vi "Configure DC Input Resistance.vi"(8 "error in (no error)":errorcluster, 10 "DC Input Resistance Mode (0: Fixed)":u16(ring) items=["Fixed", "Auto"], 11 "VISA resource name":refnum<visa-resource-name>) -> (0 "error out":errorcluster, 3 "VISA resource name out":refnum<visa-resource-name>)   [LabVIEW 2020, in "Agilent 34401.lvlib"]
doc: "Sets the input resistance for voltage readings."
uses:
  <instrlib>/Agilent 34401/Agilent 34401.lvlib
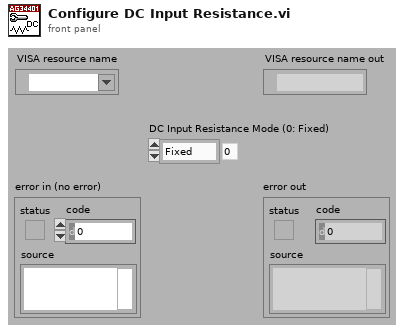
[diagram p1: front panel]
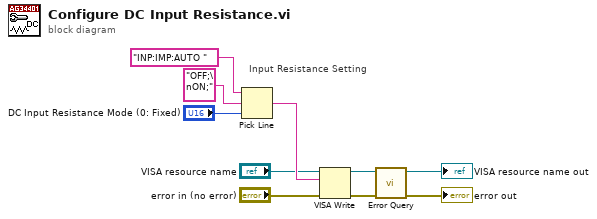
[diagram p0: block diagram]
diagram:
  # "Input Resistance Setting"
  n1 = Pick Line(string ("")="INP:IMP:AUTO ", multi-line string="OFF;\nON;", line index="DC Input Resistance Mode (0: Fixed)") -> (output string=w10:string)
  n2 = VISA Write(VISA resource name="VISA resource name", write buffer=w10, error in (no error)="error in (no error)") -> (VISA resource name out=w8:refnum<visa-resource-name>, error out=w9:errorcluster)  [unwired: 1 out]
  n3 = call <instrlib>:"Error Query.vi"("error in (no error)"=w9, "VISA resource name"=w8) -> ("error out"=→"error out":errorcluster, "VISA resource name out"=→"VISA resource name out":refnum<visa-resource-name>)  [unwired: 6 in, 2 out]
